vi "RelayOnOff.vi"   [LabVIEW 2018]
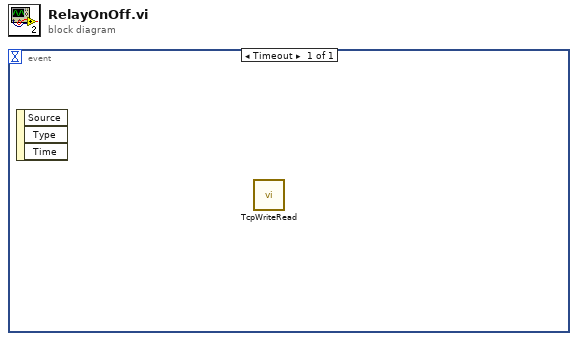
[diagram p0: block diagram]
diagram:
  n1 = event shown="[0] Timeout" {
    selector: _ -> [_]
    dyn-events: _ -> [_]
    timeout: _ -> [_]
    event Timeout {
      n2 = event-data() -> ()  [unwired: 1 in, 3 out]
      n3 = call "TcpWriteRead.vi"() -> ()  [unwired: 10 in, 2 out]
    }
  }
